vi "Clean Up Block Diagram.vi"(0 "VI Ref In":refnum<vi>, 11 "Error In":errorcluster) -> (4 "VI Ref Out":refnum<vi>, 15 "Error Out":errorcluster)   [LabVIEW 2019, in "JsonToCluster.lvlib"]
doc: "This VI cleans up block diagram for the given VI Ref"
uses:
  JsonToCluster.lvlib
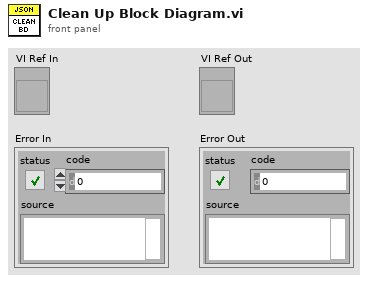
[diagram p1: front panel]
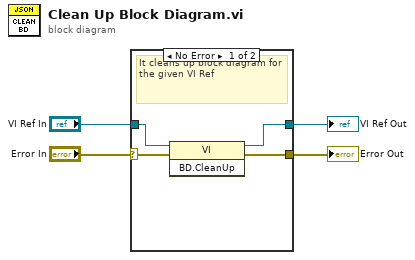
[diagram p0: block diagram]
diagram:
  n1 = case shown="No Error" "Error In" {
    selector: "Error In" -> [w8 w9]
    tunnel: [w7 w9] -> w2
    tunnel: [w6 w10] -> w3
    tunnel: "VI Ref In" -> [w5 w10]
    frame No Error {
      # "It cleans up block diagram for the given VI Ref"
      n2 = invoke class="VI" method="BD.CleanUp"(reference=w5, error in=w8) -> (reference out=w6:refnum<vi>, error out=w7:errorcluster)  [unwired: 1 in, 1 out]
    }
    frame Error {
    }
  }
  "VI Ref Out" <- w3
  "Error Out" <- w2
